vi "ADCP_write_parameter.vi"(0 "ADCP in":refnum<class "ADCP.lvclass">, 5 "Parameter Name":string, 7 "Parameter Index":i32=-1, 9 "Parameter Value":string, 11 "error in (no error)":errorcluster) -> (4 "ADCP out":refnum<class "ADCP.lvclass">, 6 "Data Packet out":T2, 15 "error out":errorcluster)   [LabVIEW 2017, in "ADCP.lvclass"]
uses:
  ADCP.lvclass
  ADCP_Data_Packet_Transmit_Mode.ctl
  ADCP.lvclass/ADCP.ctl
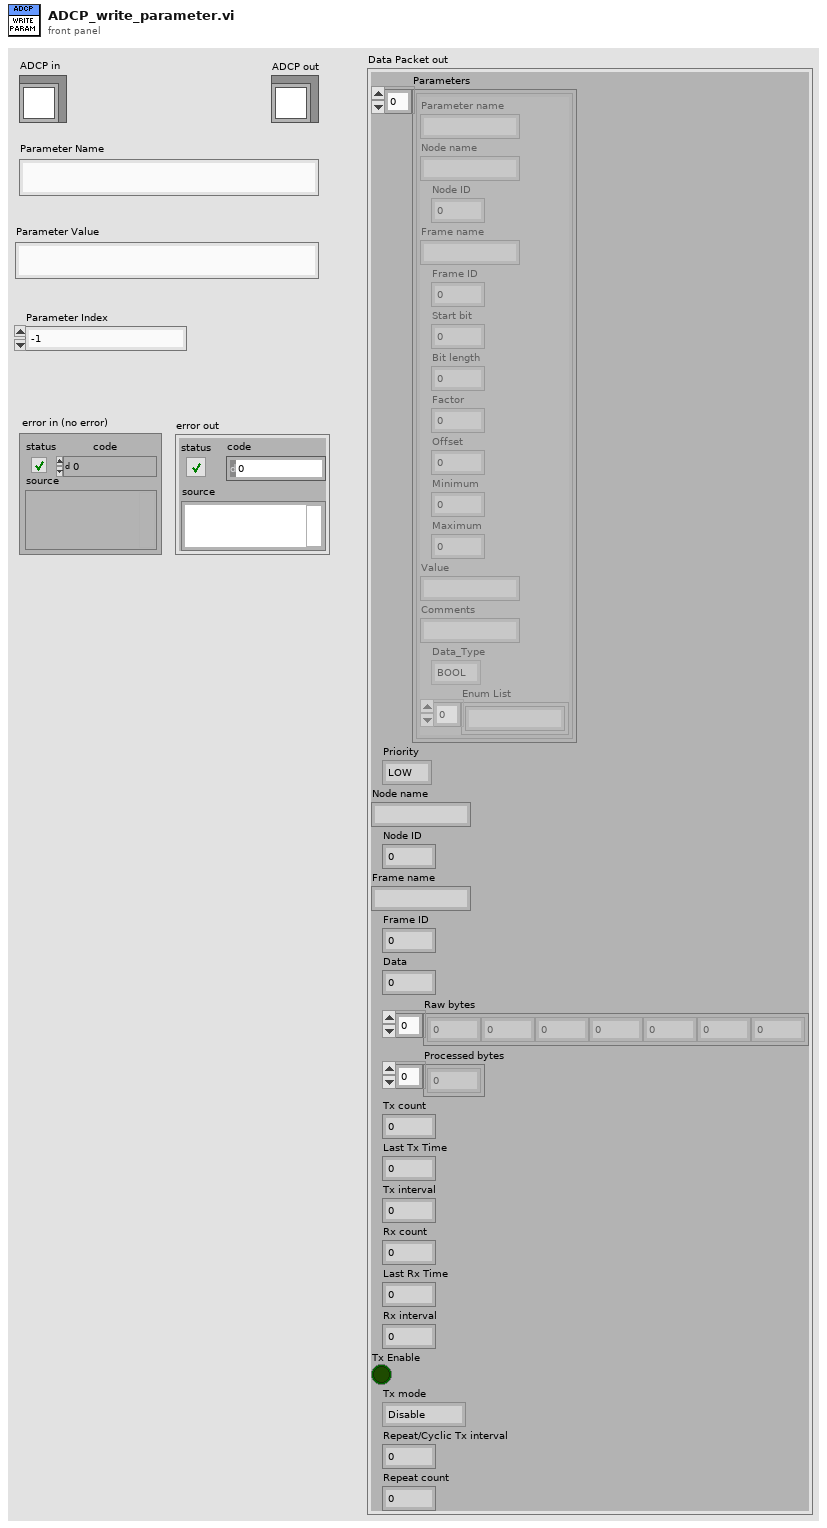
[diagram p1: front panel]
types:
  T1 = typedef "ADCP.lvclass/ADCP_Data_Packet_Transmit_Mode.ctl" = enum16{"Disable", "Single", "Cyclic", "Repeat"}
  T2 = cluster{"Parameters":cluster{"Parameter name":string, "Node name":string, "Node ID":u8, "Frame name":string, "Frame ID":u8, "Start bit":u32, "Bit length":u32, "Factor":dbl, "Offset":dbl, "Minimum":dbl, "Maximum":dbl, "Value":string, "Comments":string, "Data_Type":enum16{"BOOL", "UNSIGNED", "SIGNED", "FLOAT32", "ENUM"}, "Enum List":string[]}[], "Priority":enum16{"LOW", "HIGH"}, "Node name":string, "Node ID":u8, "Frame name":string, "Frame ID":u8, "Data":u32, "Raw bytes":u8[], "Processed bytes":u8[], "Tx count":i32, "Last Tx Time":u32, "Tx interval":u32, "Rx count":i32, "Last Rx Time":u32, "Rx interval":u32, "Tx Enable":bool, "Tx mode":T1, "Repeat/Cyclic Tx interval":u32, "Repeat count":u16}
  T3 = cluster{"Parameter name":string, "Node name":string, "Node ID":u8, "Frame name":string, "Frame ID":u8, "Start bit":u32, "Bit length":u32, "Factor":dbl, "Offset":dbl, "Minimum":dbl, "Maximum":dbl, "Value":string, "Comments":string, "Data_Type":enum16{"BOOL", "UNSIGNED", "SIGNED", "FLOAT32", "ENUM"}, "Enum List":string[]}[]
  T4 = cluster{"Parameter name":string, "Node name":string, "Node ID":u8, "Frame name":string, "Frame ID":u8, "Start bit":u32, "Bit length":u32, "Factor":dbl, "Offset":dbl, "Minimum":dbl, "Maximum":dbl, "Value":string, "Comments":string, "Data_Type":enum16{"BOOL", "UNSIGNED", "SIGNED", "FLOAT32", "ENUM"}, "Enum List":string[]}
  T5 = enum16{"BOOL", "UNSIGNED", "SIGNED", "FLOAT32", "ENUM"}
  T6 = cluster{"Parameters":cluster{"Parameter name":string, "Node name":string, "Node ID":u8, "Frame name":string, "Frame ID":u8, "Start bit":u32, "Bit length":u32, "Factor":dbl, "Offset":dbl, "Minimum":dbl, "Maximum":dbl, "Value":string, "Comments":string, "Data_Type":enum16{"BOOL", "UNSIGNED", "SIGNED", "FLOAT32", "ENUM"}, "Enum List":string[]}[], "Priority":enum16{"LOW", "HIGH"}, "Node name":string, "Node ID":u8, "Frame name":string, "Frame ID":u8, "Data":u32, "Raw bytes":u8[], "Processed bytes":u8[], "Tx count":i32, "Last Tx Time":u32, "Tx interval":u32, "Rx count":i32, "Last Rx Time":u32, "Rx interval":u32, "Tx Enable":bool, "Tx mode":T1, "Repeat/Cyclic Tx interval":u32, "Repeat count":u16}[]
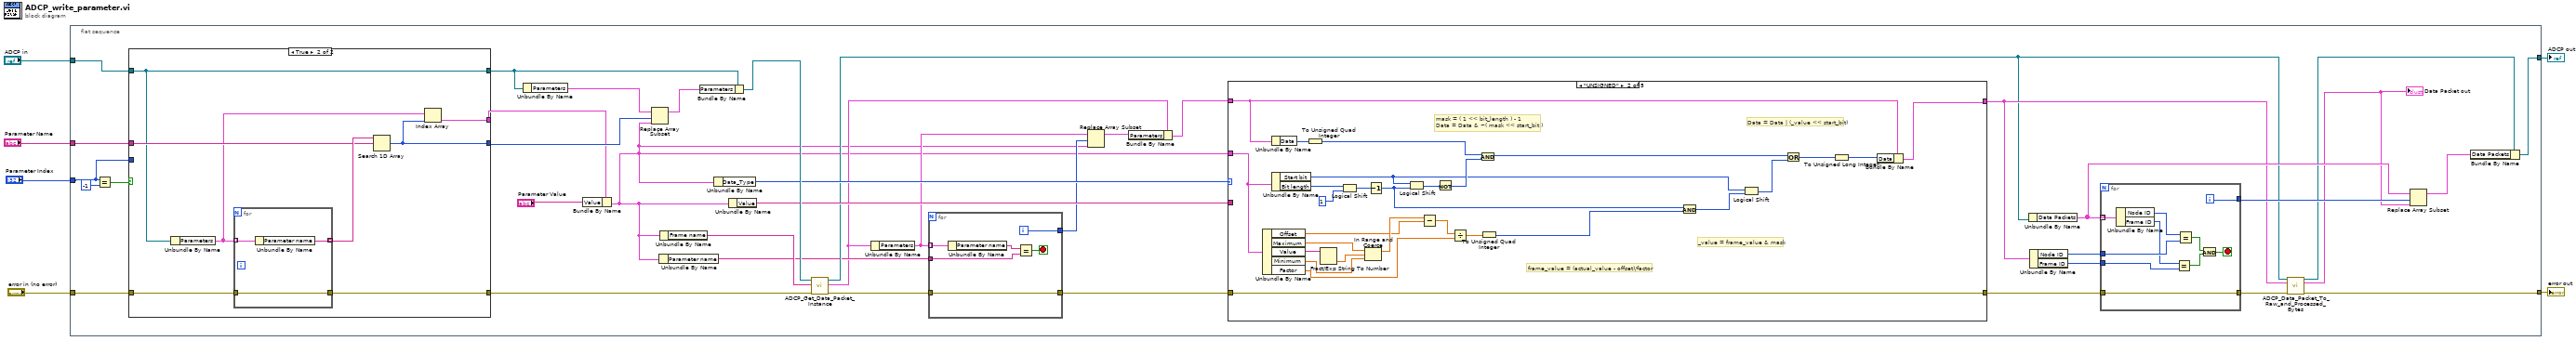
[diagram p0: block diagram]
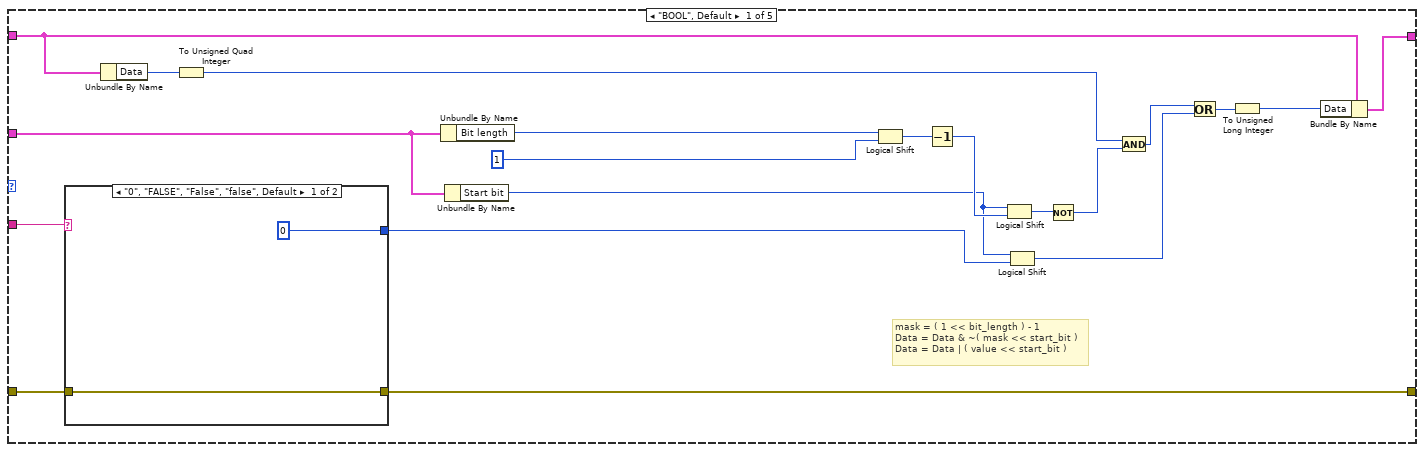
[diagram p2: hidden frame]
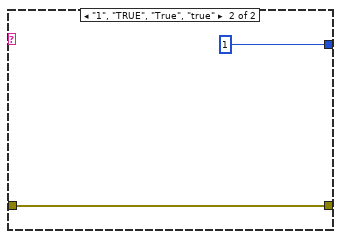
[diagram p3: hidden frame]
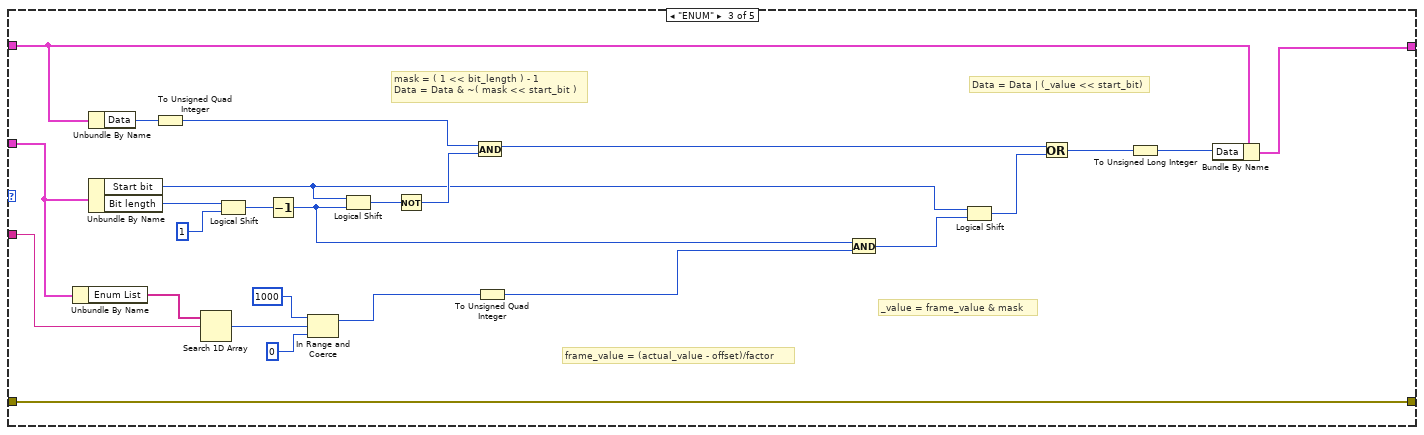
[diagram p4: hidden frame]
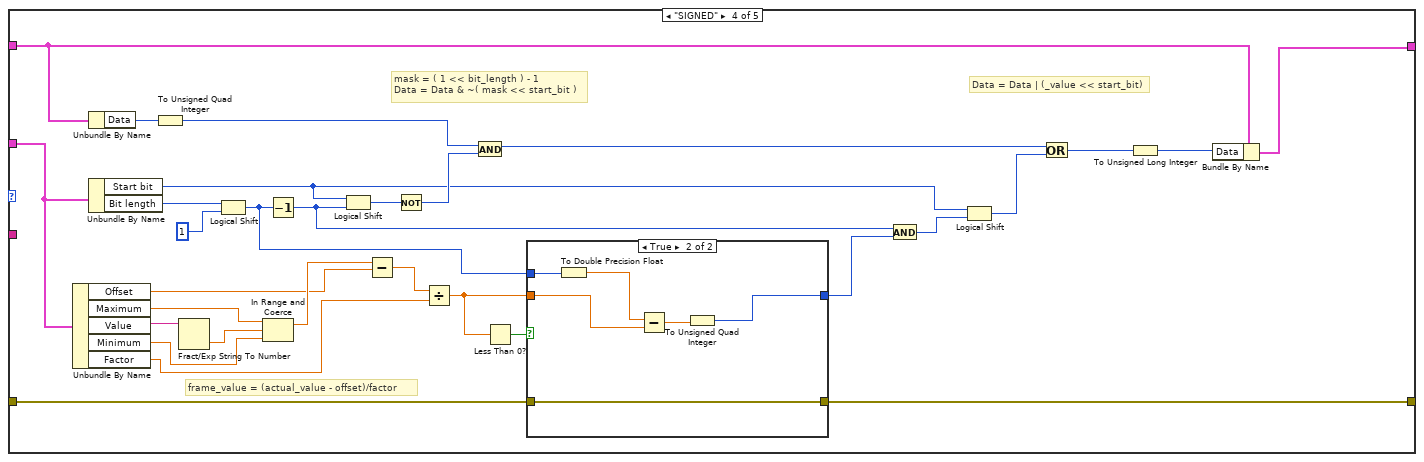
[diagram p5: hidden frame]
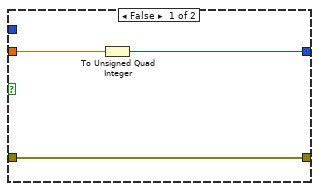
[diagram p6: hidden frame]
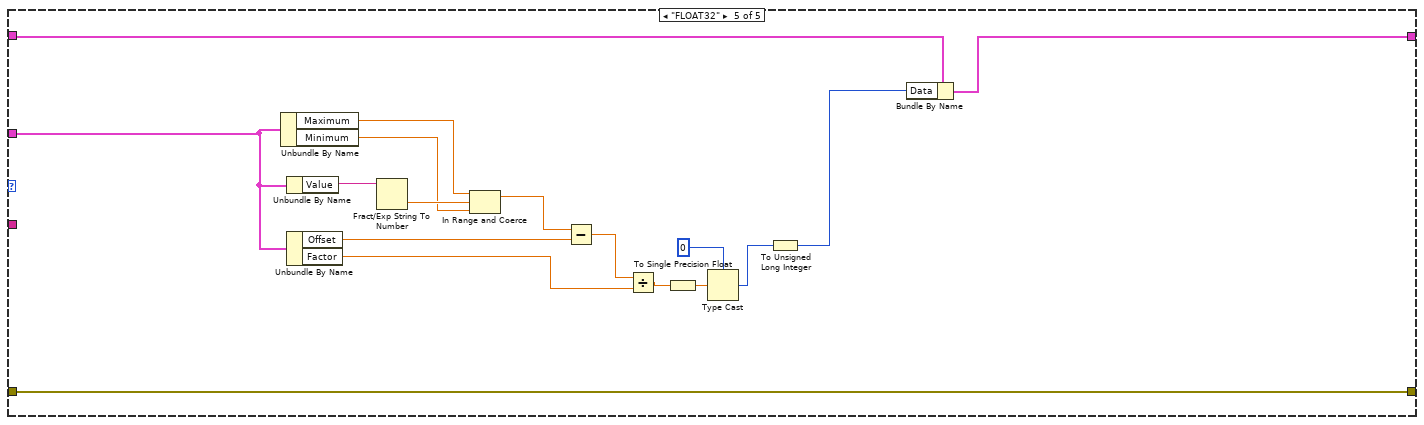
[diagram p7: hidden frame]
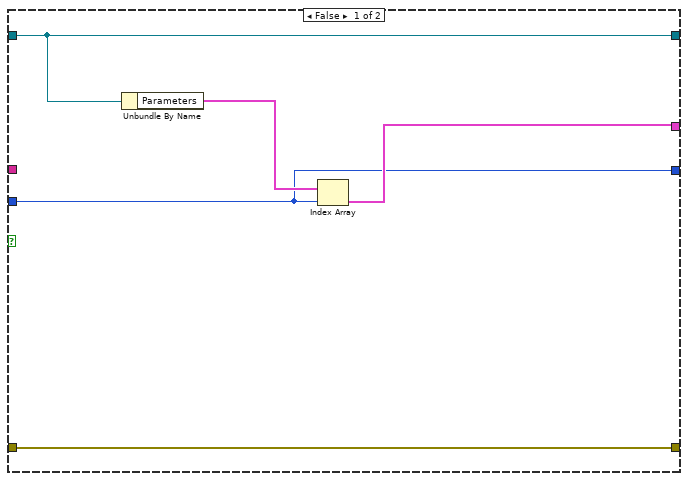
[diagram p8: hidden frame]
diagram:
  n1 = flat-sequence {
    tunnel: "error in (no error)" -> [w43]
    tunnel: "Parameter Index" -> [w40]
    tunnel: "Parameter Name" -> [w41]
    tunnel: "ADCP in" -> [w42]
    tunnel: [w22] -> w2
    tunnel: [w20] -> w1
    frame #0 {
      n2 = Equal?(x=w40, y=-1) -> (x = y?=w44:bool)
      n3 = case shown="True" w44 {
        tunnel: w43 -> [w197 w207]
        tunnel: w42 -> [w196 w201]
        tunnel: w41 -> [_ w205]
        tunnel: [w198 w203] -> w29
        tunnel: [w197 w202] -> w34
        tunnel: w40 -> [w195 _]
        tunnel: [w196 w201] -> w36
        tunnel: [w195 w200] -> w37
        frame False {
          n4 = Unbundle By Name(w196) -> ("Parameters"=w199:T3)
          n5 = Index Array(array=w199, index=w195) -> (element=w198:T4)
        }
        frame True {
          n6 = Unbundle By Name(w201) -> ("Parameters"=w204:T3)
          n7 = for {
            tunnel: w207 -> [w208]
            tunnel: w204 -> [w210] mode=indexing
            tunnel: [w209] -> w206 mode=indexing
            tunnel: [w208] -> w202
            n8 = Unbundle By Name(w210) -> ("Parameter name"=w209:string)
          }
          n9 = Search 1D Array(1D array=w206, element=w205) -> (index of element=w200:i32)  [unwired: 1 in]
          n10 = Index Array(array=w204, index=w200) -> (element=w203:T4)
        }
      }
      n11 = Unbundle By Name(w36) -> ("Parameters"=w38:T3)
      n12 = Bundle By Name(cluster=w29, "Value"="Parameter Value") -> (w7:T4)
      n13 = Replace Array Subset(array=w38, new element=w7, index=w37) -> (w35:T3)
      n14 = Unbundle By Name(w7) -> ("Parameter name"=w14:string)
      n15 = Unbundle By Name(w7) -> ("Frame name"=w32:string)
      n16 = Bundle By Name(cluster=w36, "Parameters"=w35) -> (w33:refnum<class "ADCP.lvclass">)
      n17 = Unbundle By Name(w7) -> ("Data_Type"=w31:T5)
      n18 = Unbundle By Name(w7) -> ("Value"=w30:string)
      n19 = call "ADCP_Get_Data_Packet_Instance.vi"("error in (no error)"=w34, "Frame name"=w32, "ADCP in"=w33) -> ("error out"=w15:errorcluster, "Data Packet"=w10:T2, "ADCP out"=w18:refnum<class "ADCP.lvclass">)  [unwired: 6 in]
      n20 = Unbundle By Name(w10) -> ("Parameters"=w13:T3)
      n21 = for {
        tunnel: w15 -> [w48]
        tunnel: w13 -> [w46] mode=indexing
        tunnel: w14 -> [w50]
        tunnel: [w49] -> w12
        tunnel: [w48] -> w8
        i -> [w49]
        stop <- w47 stop-if-true
        n22 = Unbundle By Name(w46) -> ("Parameter name"=w51:string)
        n23 = Equal?(x=w51, y=w50) -> (x = y?=w47:bool)
      }
      n24 = Replace Array Subset(array=w13, new element=w7, index=w12) -> (w11:T3)
      n25 = Bundle By Name(cluster=w10, "Parameters"=w11) -> (w9:T2)
      n26 = case shown="\"UNSIGNED\"" w31 {
        tunnel: w8 -> [w80 w86 w121 w144 w179]
        tunnel: w30 -> [w81 _ w118 _ _]
        tunnel: w9 -> [w65 w90 w125 w148 w181]
        tunnel: w7 -> [w75 w106 w120 w162 w182]
        tunnel: [w63 w88 w123 w146 w178] -> w19
        tunnel: [w62 w86 w121 w139 w179] -> w26
        frame "BOOL", Default {
          # "mask = ( 1 << bit_length ) - 1\nData = Data & ~( mask << start_bit )\nData = Data | ( value << start_bit )"
          n27 = case shown="\"0\", \"FALSE\", \"False\", \"false\", Default" w81 {
            tunnel: w80 -> [w83 w85]
            tunnel: [w83 w85] -> w62
            tunnel: [u64 0 u64 1] -> w69
            frame "0", "FALSE", "False", "false", Default {
            }
            frame "1", "TRUE", "True", "true" {
            }
          }
          n28 = Unbundle By Name(w65) -> ("Data"=w73:u32)
          n29 = To Unsigned Quad Integer(1:w73) -> (0:w71:u64)
          n30 = Unbundle By Name(w75) -> ("Bit length"=w79:u32)
          n31 = Unbundle By Name(w75) -> ("Start bit"=w70:u32)
          n32 = Logical Shift(y=w79, x=u64 1) -> (x << y=w77:u64)
          n33 = Decrement(x=w77) -> (x-1=w76:u64)
          n34 = Logical Shift(y=w70, x=w76) -> (x << y=w74:u64)
          n35 = Logical Shift(y=w70, x=w69) -> (x << y=w67:u64)
          n36 = Not(x=w74) -> (.not. x?=w72:u64)
          n37 = And(x=w71, y=w72) -> (x .and. y?=w68:u64)
          n38 = Or(x=w68, y=w67) -> (x .or. y?=w66:u64)
          n39 = To Unsigned Long Integer(number=w66) -> (unsigned 32bit integer=w64:u32)
          n40 = Bundle By Name(cluster=w65, "Data"=w64) -> (w63:T2)
        }
        frame "UNSIGNED" {
          # "_value = frame_value & mask"
          # "frame_value = (actual_value - offset)/factor"
          # "Data = Data | (_value << start_bit)"
          # "mask = ( 1 << bit_length ) - 1\nData = Data & ~( mask << start_bit )"
          n41 = Unbundle By Name(w106) -> ("Offset"=w100:dbl, "Maximum"=w103:dbl, "Value"=w105:string, "Minimum"=w104:dbl, "Factor"=w98:dbl)
          n42 = Unbundle By Name(w90) -> ("Data"=w113:u32)
          n43 = Unbundle By Name(w106) -> ("Start bit"=w93:u32, "Bit length"=w112:u32)
          n44 = To Unsigned Quad Integer(1:w113) -> (0:w108:u64)
          n45 = Fract/Exp String To Number(string=w105) -> (number=w102:dbl)  [unwired: 3 in, 1 out]
          n46 = Logical Shift(y=w112, x=u64 1) -> (x << y=w110:u64)
          n47 = In Range and Coerce(upper limit=w103, x=w102, lower limit=w104) -> (coerced(x)=w101:dbl)  [unwired: 1 out]
          n48 = Decrement(x=w110) -> (x-1=w95:u64)
          n49 = Logical Shift(y=w93, x=w95) -> (x << y=w109:u64)
          n50 = Subtract(x=w101, y=w100) -> (x-y=w99:dbl)
          n51 = Not(x=w109) -> (.not. x?=w107:u64)
          n52 = Divide(x=w99, y=w98) -> (x/y=w97:dbl)
          n53 = And(x=w108, y=w107) -> (x .and. y?=w92:u64)
          n54 = To Unsigned Quad Integer(1:w97) -> (0:w96:u64)
          n55 = And(x=w95, y=w96) -> (x .and. y?=w94:u64)
          n56 = Logical Shift(y=w93, x=w94) -> (x << y=w91:u64)
          n57 = Or(x=w92, y=w91) -> (x .or. y?=w89:u64)
          n58 = To Unsigned Long Integer(number=w89) -> (unsigned 32bit integer=w87:u32)
          n59 = Bundle By Name(cluster=w90, "Data"=w87) -> (w88:T2)
        }
        frame "ENUM" {
          # "_value = frame_value & mask"
          # "frame_value = (actual_value - offset)/factor"
          # "Data = Data | (_value << start_bit)"
          # "mask = ( 1 << bit_length ) - 1\nData = Data & ~( mask << start_bit )"
          n60 = Unbundle By Name(w120) -> ("Enum List"=w119:string[])
          n61 = Unbundle By Name(w125) -> ("Data"=w138:u32)
          n62 = Unbundle By Name(w120) -> ("Start bit"=w128:u32, "Bit length"=w137:u32)
          n63 = To Unsigned Quad Integer(1:w138) -> (0:w133:u64)
          n64 = Search 1D Array(1D array=w119, element=w118) -> (index of element=w117:i32)  [unwired: 1 in]
          n65 = Logical Shift(y=w137, x=u64 1) -> (x << y=w135:u64)
          n66 = Decrement(x=w135) -> (x-1=w130:u64)
          n67 = In Range and Coerce(upper limit=1000, x=w117, lower limit=0) -> (coerced(x)=w114:i32)  [unwired: 1 out]
          n68 = Logical Shift(y=w128, x=w130) -> (x << y=w134:u64)
          n69 = Not(x=w134) -> (.not. x?=w132:u64)
          n70 = And(x=w133, y=w132) -> (x .and. y?=w127:u64)
          n71 = To Unsigned Quad Integer(1:w114) -> (0:w131:u64)
          n72 = And(x=w130, y=w131) -> (x .and. y?=w129:u64)
          n73 = Logical Shift(y=w128, x=w129) -> (x << y=w126:u64)
          n74 = Or(x=w127, y=w126) -> (x .or. y?=w124:u64)
          n75 = To Unsigned Long Integer(number=w124) -> (unsigned 32bit integer=w122:u32)
          n76 = Bundle By Name(cluster=w125, "Data"=w122) -> (w123:T2)
        }
        frame "SIGNED" {
          # "frame_value = (actual_value - offset)/factor"
          # "Data = Data | (_value << start_bit)"
          # "mask = ( 1 << bit_length ) - 1\nData = Data & ~( mask << start_bit )"
          n77 = Unbundle By Name(w162) -> ("Offset"=w156:dbl, "Maximum"=w159:dbl, "Value"=w161:string, "Minimum"=w160:dbl, "Factor"=w154:dbl)
          n78 = Unbundle By Name(w148) -> ("Data"=w168:u32)
          n79 = Unbundle By Name(w162) -> ("Start bit"=w151:u32, "Bit length"=w167:u32)
          n80 = To Unsigned Quad Integer(1:w168) -> (0:w164:u64)
          n81 = Fract/Exp String To Number(string=w161) -> (number=w158:dbl)  [unwired: 3 in, 1 out]
          n82 = Logical Shift(y=w167, x=u64 1) -> (x << y=w140:u64)
          n83 = In Range and Coerce(upper limit=w159, x=w158, lower limit=w160) -> (coerced(x)=w157:dbl)  [unwired: 1 out]
          n84 = Decrement(x=w140) -> (x-1=w153:u64)
          n85 = Logical Shift(y=w151, x=w153) -> (x << y=w165:u64)
          n86 = Subtract(x=w157, y=w156) -> (x-y=w155:dbl)
          n87 = Not(x=w165) -> (.not. x?=w163:u64)
          n88 = Divide(x=w155, y=w154) -> (x/y=w142:dbl)
          n89 = And(x=w164, y=w163) -> (x .and. y?=w150:u64)
          n90 = Less Than 0?(x=w142) -> (x < 0?=w143:bool)
          n91 = case shown="True" w143 {
            tunnel: w144 -> [w169 w172]
            tunnel: w142 -> [w171 w175]
            tunnel: [w170 w173] -> w141
            tunnel: w140 -> [_ w177]
            tunnel: [w169 w172] -> w139
            frame False {
              n92 = To Unsigned Quad Integer(1:w171) -> (0:w170:u64)
            }
            frame True {
              n93 = To Double Precision Float(number=w177) -> (double precision float=w176:dbl)
              n94 = Subtract(x=w176, y=w175) -> (x-y=w174:dbl)
              n95 = To Unsigned Quad Integer(1:w174) -> (0:w173:u64)
            }
          }
          n96 = And(x=w153, y=w141) -> (x .and. y?=w152:u64)
          n97 = Logical Shift(y=w151, x=w152) -> (x << y=w149:u64)
          n98 = Or(x=w150, y=w149) -> (x .or. y?=w147:u64)
          n99 = To Unsigned Long Integer(number=w147) -> (unsigned 32bit integer=w145:u32)
          n100 = Bundle By Name(cluster=w148, "Data"=w145) -> (w146:T2)
        }
        frame "FLOAT32" {
          n101 = Unbundle By Name(w182) -> ("Maximum"=w189:dbl, "Minimum"=w188:dbl)
          n102 = Unbundle By Name(w182) -> ("Value"=w194:string)
          n103 = Unbundle By Name(w182) -> ("Offset"=w193:dbl, "Factor"=w191:dbl)
          n104 = Fract/Exp String To Number(string=w194) -> (number=w190:dbl)  [unwired: 3 in, 1 out]
          n105 = In Range and Coerce(upper limit=w189, x=w190, lower limit=w188) -> (coerced(x)=w187:dbl)  [unwired: 1 out]
          n106 = Subtract(x=w187, y=w193) -> (x-y=w192:dbl)
          n107 = Divide(x=w192, y=w191) -> (x/y=w186:dbl)
          n108 = To Single Precision Float(number=w186) -> (single precision float=w185:sgl)
          n109 = Type Cast(type=u32 0, x=w185) -> (*(type *) &x=w183:u32)
          n110 = To Unsigned Long Integer(number=w183) -> (unsigned 32bit integer=w180:u32)
          n111 = Bundle By Name(cluster=w181, "Data"=w180) -> (w178:T2)
        }
      }
      n112 = Unbundle By Name(w18) -> ("Data Packets"=w25:T6)
      n113 = Unbundle By Name(w19) -> ("Node ID"=w28:u8, "Frame ID"=w27:u8)
      n114 = for {
        tunnel: w25 -> [w52] mode=indexing
        tunnel: w28 -> [w60]
        tunnel: w27 -> [w58]
        tunnel: [w55] -> w24
        tunnel: w26 -> [w53]
        tunnel: [w53] -> w21
        i -> [w55]
        stop <- w54 stop-if-true
        n115 = Unbundle By Name(w52) -> ("Node ID"=w61:u8, "Frame ID"=w59:u8)
        n116 = Equal?(x=w59, y=w58) -> (x = y?=w56:bool)
        n117 = Equal?(x=w61, y=w60) -> (x = y?=w57:bool)
        n118 = And(x=w57, y=w56) -> (x .and. y?=w54:bool)
      }
      n119 = call "ADCP_Data_Packet_To_Raw_and_Processed_Bytes.vi"("ADCP In"=w18, "Data Packet In"=w19, "error in (no error)"=w21) -> ("ADCP out"=w17:refnum<class "ADCP.lvclass">, "Data Packet out"=w16:T2, "error out"=w20:errorcluster)  [unwired: 8 in, 2 out]
      "Data Packet out" <- w16
      n120 = Replace Array Subset(array=w25, new element=w16, index=w24) -> (w23:T6)
      n121 = Bundle By Name(cluster=w17, "Data Packets"=w23) -> (w22:refnum<class "ADCP.lvclass">)
    }
  }
  "ADCP out" <- w2
  "error out" <- w1
